vi "LowerSwitchPressed.vi"() -> ()   [LabVIEW 2017]
panel:
  out "SwitchPressedLow":bool
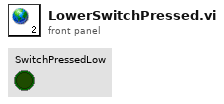
[diagram p1: front panel]
diagram:
